vi "C3--cube Sw.vi"(8 "Command Info In":T1, 10 "C3--cube Sw":T4, 11 "Switch":string) -> (0 "Command Info Out":T1)   [LabVIEW 2017]
uses:
  <vilib>/Rock Robotics/WPI/Framework/Command Status Info.ctl
  <vilib>/Rock Robotics/WPI/Framework/Completion Status.ctl
  <vilib>/Rock Robotics/WPI/Framework/Completion Notifier.ctl
  Block Clusters/C3--cube Sw.ctl
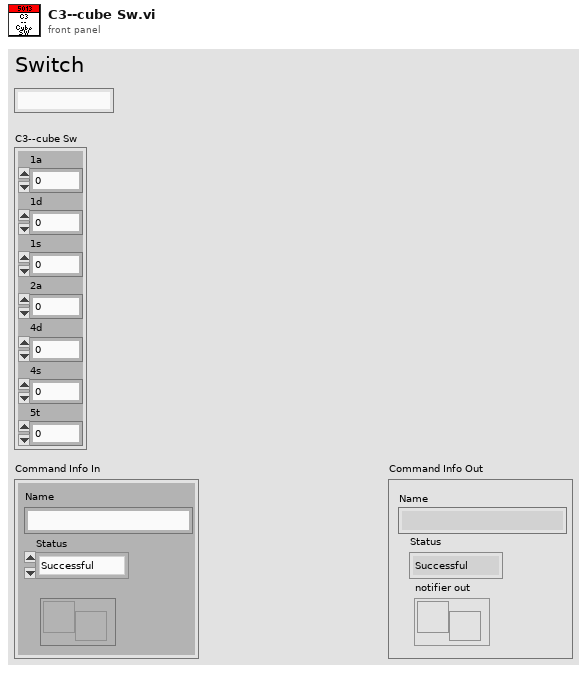
[diagram p1: front panel]
types:
  T1 = typedef "Command Status Info.ctl" = cluster{"Name":string, "Status":T2, "notifier out":T3}
  T2 = typedef "Completion Status.ctl" = enum16{"Successful", "Aborted", "Incomplete"}
  T3 = typedef "Completion Notifier.ctl" = refnum<notifier>
  T4 = typedef "C3--cube Sw.ctl" = cluster{"1a":dbl, "1d":dbl, "1s":dbl, "2a":dbl, "4d":dbl, "4s":dbl, "5t":dbl}
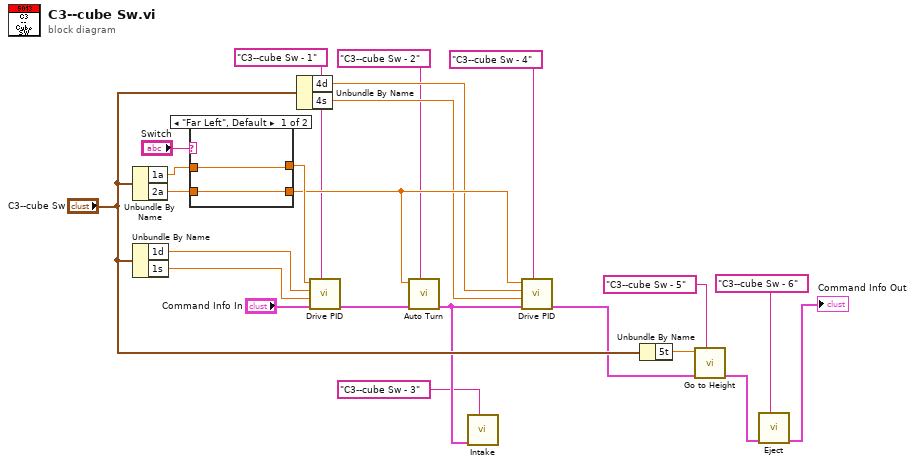
[diagram p0: block diagram]
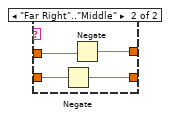
[diagram p2: hidden frame]
diagram:
  n1 = Unbundle By Name("C3--cube Sw") -> ("1a"=w10:dbl, "2a"=w9:dbl)
  n2 = Unbundle By Name("C3--cube Sw") -> ("1d"=w19:dbl, "1s"=w18:dbl)
  n3 = case shown="\"Far Left\", Default" "Switch" {
    tunnel: [w25 w29] -> w20
    tunnel: w10 -> [w25 w28]
    tunnel: w9 -> [w24 w27]
    tunnel: [w24 w26] -> w17
    frame "Far Left", Default {
    }
    frame "Far Right".."Middle" {
      n4 = Negate(x=w27) -> (-x=w26:dbl)
      n5 = Negate(x=w28) -> (-x=w29:dbl)
    }
  }
  n6 = Unbundle By Name("C3--cube Sw") -> ("4d"=w16:dbl, "4s"=w15:dbl)
  n7 = call "Drive PID.vi"("Description"="C3--cube Sw - 1", "Command Info In"="Command Info In", "Speed"=w18, "Distance"=w19, "Target Angle"=w20) -> ("Command Info Out"=w22:T1)  [unwired: 6 in]
  n8 = call "Auto Turn.vi"("Description"="C3--cube Sw - 2", "Command Info In"=w22, "Target Angle"=w17) -> ("Command Info Out"=w6:T1)  [unwired: 8 in]
  n9 = call "Intake.vi"("Description"="C3--cube Sw - 3", "Command Info In"=w6) -> ()  [unwired: 9 in, 1 out]
  n10 = call "Drive PID.vi"("Description"="C3--cube Sw - 4", "Command Info In"=w6, "Speed"=w15, "Distance"=w16, "Target Angle"=w17) -> ("Command Info Out"=w5:T1)  [unwired: 6 in]
  n11 = Unbundle By Name("C3--cube Sw") -> ("5t"=w14:dbl)
  n12 = call "Go to Height.vi"("Description"="C3--cube Sw - 5", "Command Info In"=w5, "Target Height (in)"=w14) -> ("Command Info Out"=w21:T1)  [unwired: 8 in]
  n13 = call "Eject.vi"("Description"="C3--cube Sw - 6", "Command Info In"=w21) -> ("Command Info Out"=→"Command Info Out":T1)  [unwired: 9 in]
